vi "Get Intermediate String.vi"(1 "End Delimiter":string, 2 "Input String":string, 3 "Start Delimiter":string) -> (0 "Output String":string)   [LabVIEW 2021]
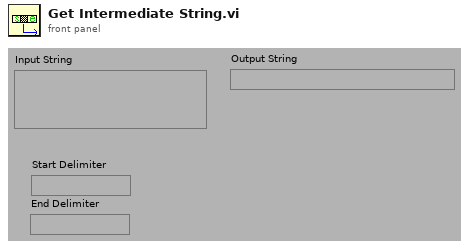
[diagram p1: front panel]
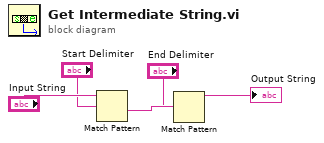
[diagram p0: block diagram]
diagram:
  n1 = Match Pattern(string="Input String", regular expression="Start Delimiter") -> (after substring=w3:string)  [unwired: 1 in, 3 out]
  n2 = Match Pattern(string=w3, regular expression="End Delimiter") -> (before substring=→"Output String":string)  [unwired: 1 in, 3 out]
